vi "Read Dashboard Variables.vi"() -> ()   [LabVIEW 2020]
uses:
  <vilib>/Rock Robotics/Network Tables/NT Read Number.vi
  Framework/Robot Global Data.vi
  <vilib>/Rock Robotics/Network Tables/NT Read String.vi
panel:
  out "Intake Sped Up Setpoint":dbl=0.8 format="%#_13g"
  out "Intake Sped Up Duration":dbl=3.0 format="%#_13g"
  out "Custom MaxSpeedSlow (0.6)":dbl=0.6
  out "Transfer Release Duration":dbl
  out "Transfer Up Duration":dbl
  out "Pivot Duration":dbl
  out "Pivot Right Speed":dbl
  out "Pivot Left Speed":dbl
  out "Transfer Release Setpoint":dbl
  out "Transfer Up Setpoint":dbl
  out "Intake Setpoint":dbl=0.8 format="%#_13g"
  out "Intake Duration (s)":dbl=3.0 format="%#_13g"
  out "Shooter Duration (s)":dbl=3.0 format="%#_13g"
  out "Shooter Setpoint":dbl=0.8 format="%#_13g"
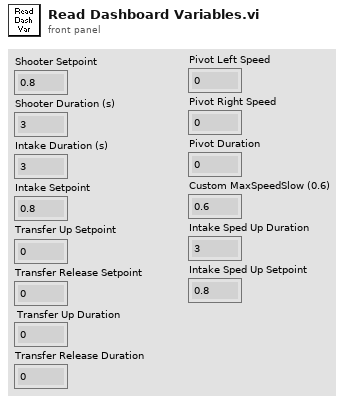
[diagram p1: front panel]
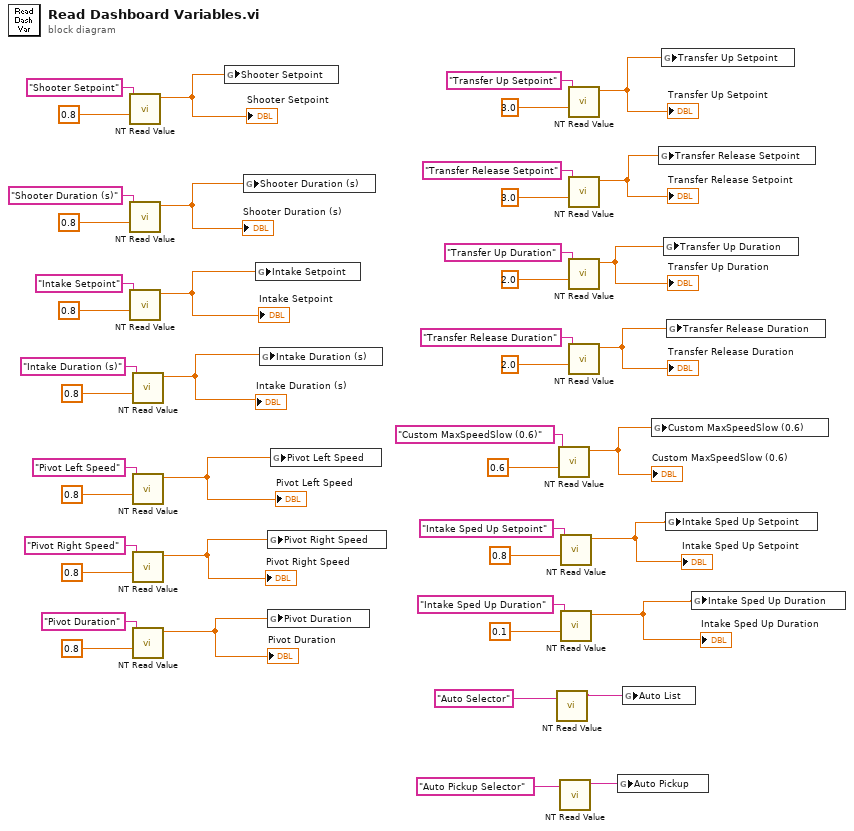
[diagram p0: block diagram]
diagram:
  n1 = call-poly <vilib>:"NT Read Value.vi"("Default Value"=0.8, "Name"="Shooter Setpoint") -> ("Numeric"=w44:dbl)  [unwired: 8 in, 1 out]
  "Shooter Setpoint" <- w44
  n2 = call-poly <vilib>:"NT Read Value.vi"("Default Value"=0.8, "Name"="Shooter Duration (s)") -> ("Numeric"=w41:dbl)  [unwired: 8 in, 1 out]
  "Shooter Duration (s)" <- w41
  n3 = call-poly <vilib>:"NT Read Value.vi"("Default Value"=0.8, "Name"="Intake Setpoint") -> ("Numeric"=w36:dbl)  [unwired: 8 in, 1 out]
  "Intake Setpoint" <- w36
  n4 = call-poly <vilib>:"NT Read Value.vi"("Default Value"=0.8, "Name"="Intake Duration (s)") -> ("Numeric"=w35:dbl)  [unwired: 8 in, 1 out]
  "Intake Duration (s)" <- w35
  n5 = call-poly <vilib>:"NT Read Value.vi"("Default Value"=0.8, "Name"="Pivot Left Speed") -> ("Numeric"=w24:dbl)  [unwired: 8 in, 1 out]
  "Pivot Left Speed" <- w24
  n6 = call-poly <vilib>:"NT Read Value.vi"("Default Value"=0.8, "Name"="Pivot Right Speed") -> ("Numeric"=w25:dbl)  [unwired: 8 in, 1 out]
  "Pivot Right Speed" <- w25
  n7 = call-poly <vilib>:"NT Read Value.vi"("Default Value"=0.8, "Name"="Pivot Duration") -> ("Numeric"=w26:dbl)  [unwired: 8 in, 1 out]
  "Pivot Duration" <- w26
  n8 = global write "Robot Global Data.vi" "Shooter Setpoint"(w44) -> ()
  n9 = global write "Robot Global Data.vi" "Shooter Duration (s)"(w41) -> ()
  n10 = global write "Robot Global Data.vi" "Intake Setpoint"(w36) -> ()
  n11 = global write "Robot Global Data.vi" "Intake Duration (s)"(w35) -> ()
  n12 = global write "Robot Global Data.vi" "Pivot Right Speed"(w25) -> ()
  n13 = global write "Robot Global Data.vi" "Pivot Duration"(w26) -> ()
  n14 = global write "Robot Global Data.vi" "Pivot Left Speed"(w24) -> ()
  n15 = call-poly <vilib>:"NT Read Value.vi"("Name"="Auto Selector") -> ("String"=w11:string)  [unwired: 9 in, 1 out]
  n16 = call-poly <vilib>:"NT Read Value.vi"("Default Value"=0.6, "Name"="Custom MaxSpeedSlow (0.6)") -> ("Numeric"=w7:dbl)  [unwired: 8 in, 1 out]
  "Custom MaxSpeedSlow (0.6)" <- w7
  n17 = call-poly <vilib>:"NT Read Value.vi"("Name"="Auto Pickup Selector") -> ("String"=w10:string)  [unwired: 9 in, 1 out]
  n18 = call-poly <vilib>:"NT Read Value.vi"("Default Value"=0.8, "Name"="Intake Sped Up Setpoint") -> ("Numeric"=w2:dbl)  [unwired: 8 in, 1 out]
  "Intake Sped Up Setpoint" <- w2
  n19 = call-poly <vilib>:"NT Read Value.vi"("Default Value"=0.1, "Name"="Intake Sped Up Duration") -> ("Numeric"=w1:dbl)  [unwired: 8 in, 1 out]
  "Intake Sped Up Duration" <- w1
  n20 = call-poly <vilib>:"NT Read Value.vi"("Default Value"=3.0, "Name"="Transfer Up Setpoint") -> ("Numeric"=w17:dbl)  [unwired: 8 in, 1 out]
  "Transfer Up Setpoint" <- w17
  n21 = call-poly <vilib>:"NT Read Value.vi"("Default Value"=3.0, "Name"="Transfer Release Setpoint") -> ("Numeric"=w16:dbl)  [unwired: 8 in, 1 out]
  "Transfer Release Setpoint" <- w16
  n22 = call-poly <vilib>:"NT Read Value.vi"("Default Value"=2.0, "Name"="Transfer Up Duration") -> ("Numeric"=w14:dbl)  [unwired: 8 in, 1 out]
  "Transfer Up Duration" <- w14
  n23 = call-poly <vilib>:"NT Read Value.vi"("Default Value"=2.0, "Name"="Transfer Release Duration") -> ("Numeric"=w15:dbl)  [unwired: 8 in, 1 out]
  "Transfer Release Duration" <- w15
  n24 = global write "Robot Global Data.vi" "Auto Pickup"(w10) -> ()
  n25 = global write "Robot Global Data.vi" "Auto List"(w11) -> ()
  n26 = global write "Robot Global Data.vi" "Custom MaxSpeedSlow (0.6)"(w7) -> ()
  n27 = global write "Robot Global Data.vi" "Transfer Release Setpoint"(w16) -> ()
  n28 = global write "Robot Global Data.vi" "Transfer Up Setpoint"(w17) -> ()
  n29 = global write "Robot Global Data.vi" "Transfer Up Duration"(w14) -> ()
  n30 = global write "Robot Global Data.vi" "Intake Sped Up Setpoint"(w2) -> ()
  n31 = global write "Robot Global Data.vi" "Transfer Release Duration"(w15) -> ()
  n32 = global write "Robot Global Data.vi" "Intake Sped Up Duration"(w1) -> ()
